vi "Agilent E3647 Dual Output.vi"(8 "error in (no error)":errorcluster, 10 "Set Command Voltage":string="VOLT:PROT:STATE ON;:VOLT:PROT 10.000000;:INST:SEL OUT1;:VOLT 3.300000;:CURR 0.006000;:INST:SEL OUT2;:VOLT 1.800000;:CURR 0.006000", 11 "VISA resource name":refnum<visa-resource-name>) -> (0 "error out":errorcluster, 3 "VISA resource name out":refnum<visa-resource-name>)   [LabVIEW 2009]
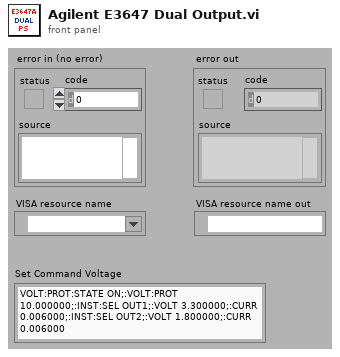
[diagram p1: front panel]
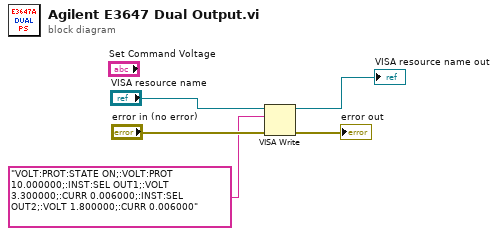
[diagram p0: block diagram]
diagram:
  n1 = VISA Write(VISA resource name="VISA resource name", write buffer="VOLT:PROT:STATE ON;:VOLT:PROT 10.000000;:INST:SEL OUT1;:VOLT 3.300000;:CURR 0.006000;:INST:SEL OUT2;:VOLT 1.800000;:CURR 0.006000", error in (no error)="error in (no error)") -> (VISA resource name out=→"VISA resource name out":refnum<visa-resource-name>, error out=→"error out":errorcluster)  [unwired: 1 out]
